vi "Generate_Complex_waveform.vi"() -> ()   [LabVIEW 2019, in "mmW_commands.lvlib"]
uses:
  mmW_commands.lvlib
  <vilib>/measure/maspectr.llb/FFT Power Spectrum and PSD for 1 Chan (CDB).vi
  <vilib>/Analysis/NI_AALBase.lvlib
  <vilib>/measure/NI_MAPro.lvlib
panel:
  out "Re":string
  out "Im":string
  out "max value":dbl
  out "x/y":dbl[](array[numeric])
  out "16bit integer":i16[](array[numeric])
  out "x+y":dbl[](array[numeric])
  out "Power Spectrum / PSD 2":cluster{"f0":dbl, "df":dbl, "magnitude":dbl[]}(graph)
  in  "Noise":dbl(slide)=1.0 scale=0.0..1.0
  out "Power Spectrum / PSD":cluster{"f0":dbl, "df":dbl, "magnitude":dbl[]}(graph)
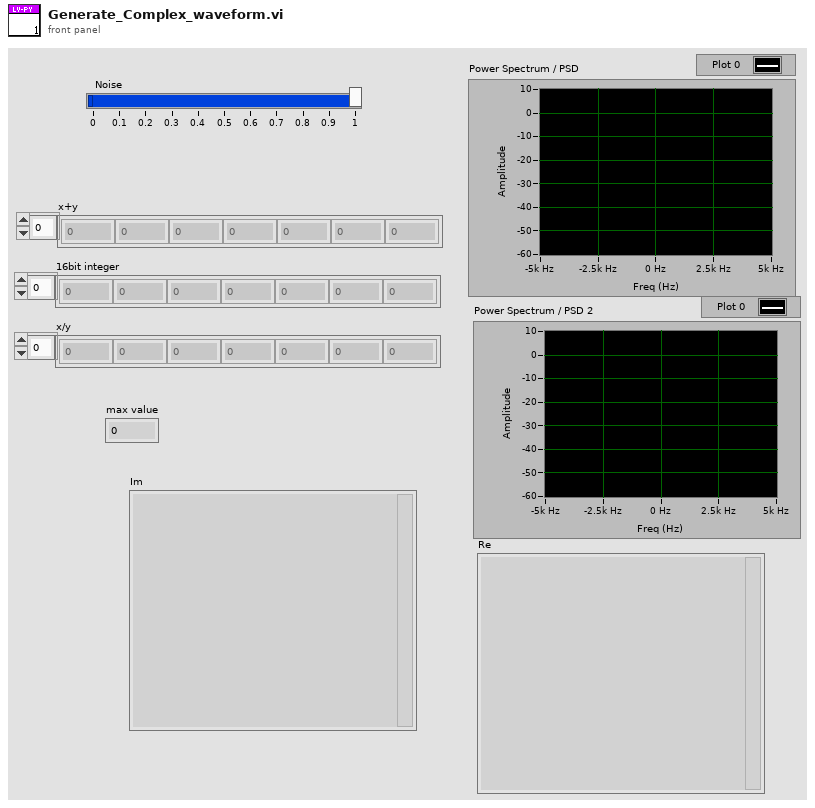
[diagram p1: front panel]
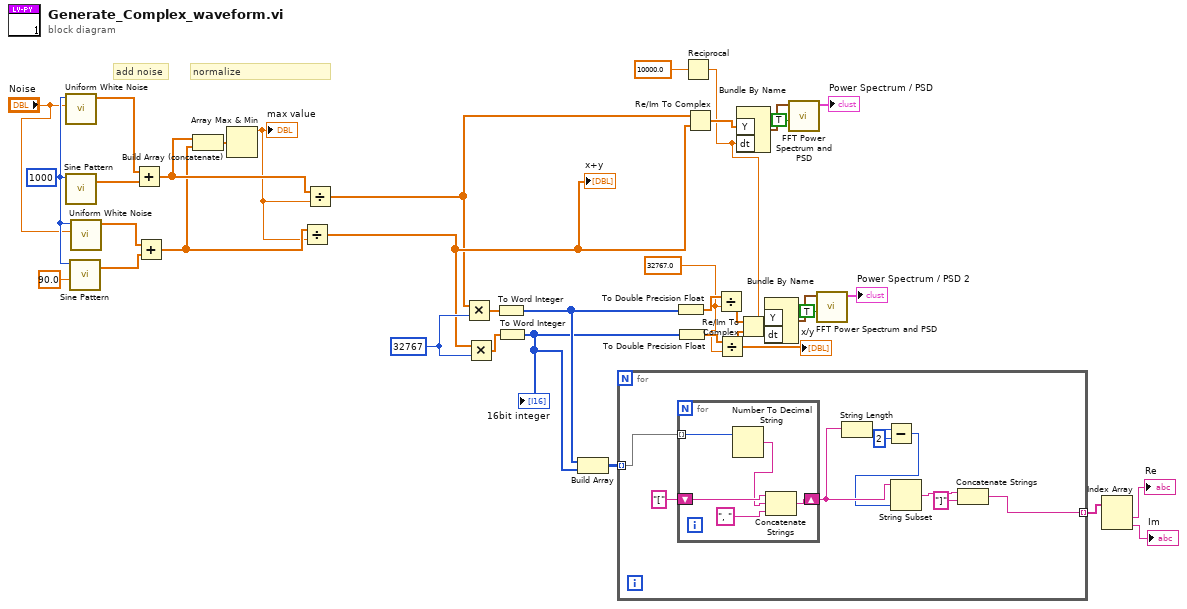
[diagram p0: block diagram]
diagram:
  w22 = 32767.0
  w36 = i16 32767
  w26 = 1000 ("samples")
  # "normalize"
  # "add noise"
  n1 = call <vilib>:"Uniform White Noise.vi"("amplitude"="Noise", "samples"=w26) -> ("uniform white noise"=w28:dbl[])  [unwired: 8 in, 1 out]
  n2 = call <vilib>:"Sine Pattern.vi"("samples"=w26) -> ("Sinusoidal Pattern"=w29:dbl[])  [unwired: 3 in, 1 out]
  n3 = call <vilib>:"Sine Pattern.vi"("phase(degrees)"=90.0, "samples"=w26) -> ("Sinusoidal Pattern"=w27:dbl[])  [unwired: 2 in, 1 out]
  n4 = call <vilib>:"Uniform White Noise.vi"("amplitude"="Noise", "samples"=w26) -> ("uniform white noise"=w25:dbl[])  [unwired: 8 in, 1 out]
  n5 = Add(x=w28, y=w29) -> (x+y=w12:dbl[])
  n6 = Add(x=w25, y=w27) -> (x+y=w11:dbl[])
  n7 = Build Array (concatenate)(w12, w11) -> (w15:dbl[])
  n8 = Array Max & Min(array=w15) -> (max value=w10:dbl)  [unwired: 3 out]
  "max value" <- w10
  n9 = Divide(x=w11, y=w10) -> (x/y=w9:dbl[])
  "x+y" <- w9
  n10 = Divide(x=w12, y=w10) -> (x/y=w8:dbl[])
  n11 = Multiply(x=w8, y=w36) -> (x*y=w35:dbl[])
  n12 = Multiply(x=w9, y=w36) -> (x*y=w34:dbl[])
  n13 = To Word Integer(number=w35) -> (16bit integer=w7:i16[])
  n14 = To Word Integer(number=w34) -> (16bit integer=w6:i16[])
  "16bit integer" <- w6
  n15 = Build Array(w7, w6) -> (w5:i16[][])
  n16 = for {
    tunnel: w5 -> [w38] mode=indexing
    tunnel: [w39] -> w4 mode=indexing
    n17 = for {
      tunnel: w38 -> [w50] mode=indexing
      shift-right: [w49] -> w43
      shift-left: "[" -> [w51]
      n18 = Number To Decimal String(number=w50) -> (decimal integer string=w48:string)  [unwired: 1 in]
      n19 = Concatenate Strings(w51, w48, ", " ("string")) -> (w49:string)
    }
    n20 = String Length(string=w43) -> (length=w45:i32)
    n21 = Subtract(x=w45, y=2) -> (x-y=w42:i32)
    n22 = String Subset(string=w43, length (rest)=w42) -> (substring=w41:string)  [unwired: 1 in]
    n23 = Concatenate Strings(w41, "]" ("string")) -> (w39:string)
  }
  n24 = To Double Precision Float(number=w7) -> (double precision float=w24:dbl[])
  n25 = To Double Precision Float(number=w6) -> (double precision float=w23:dbl[])
  n26 = Reciprocal(x=10000.0) -> (1/x=w17:dbl)
  n27 = Re/Im To Complex(1:w9, 2:w8) -> (0:w33:cdb[])
  n28 = Divide(x=w24, y=w22) -> (x/y=w19:dbl[])
  n29 = Divide(x=w23, y=w22) -> (x/y=w18:dbl[])
  "x/y" <- w18
  n30 = Bundle By Name("Y"=w33, "dt"=w17) -> (w32:waveform(cdb))  [unwired: 1 in]
  n31 = Re/Im To Complex(1:w18, 2:w19) -> (0:w16:cdb[])
  n32 = Bundle By Name("Y"=w16, "dt"=w17) -> (w20:waveform(cdb))  [unwired: 1 in]
  n33 = call-poly <vilib>:"FFT Power Spectrum and PSD.vi"("dB On (F)"=TRUE, "time signal"=w32) -> ("Power Spectrum / PSD"=→"Power Spectrum / PSD":cluster{"f0":dbl, "df":dbl, "magnitude":dbl[]})  [unwired: 6 in, 3 out]
  n34 = call-poly <vilib>:"FFT Power Spectrum and PSD.vi"("dB On (F)"=TRUE, "time signal"=w20) -> ("Power Spectrum / PSD"=→"Power Spectrum / PSD 2":cluster{"f0":dbl, "df":dbl, "magnitude":dbl[]})  [unwired: 6 in, 3 out]
  n35 = Index Array(array=w4) -> (element #1=→"Re":string, element #2=→"Im":string)  [unwired: 2 in]
